vi "FTP Move_Status_Errors.vi"(8 "error in (no error)":errorcluster, 9 "Dir of file to FTP":path, 10 "FTP input cluster":T1={"Host"="", "UserName"="", "PassWord"="", "FTP File Path"="", "Timeout (S)"=0, "ActivePasive"=FALSE, "Binary Ascii"=FALSE, "Remote Port"=21} {"Timeout (S)" min=0 max=300 step=1}, 11 "File to Move":string) -> (1 "concatenated string of Error":string, 3 "FTP completed (true = good)":bool)   [LabVIEW 2011]
uses:
  Controls/FTP Credintials.ctl
  <vilib>/addons/internet/NI_InternetTK_FTP_VIs.lvlib
panel:
  # "Passive"
  # "Active"
  # "Binary"
  # "Ascii"
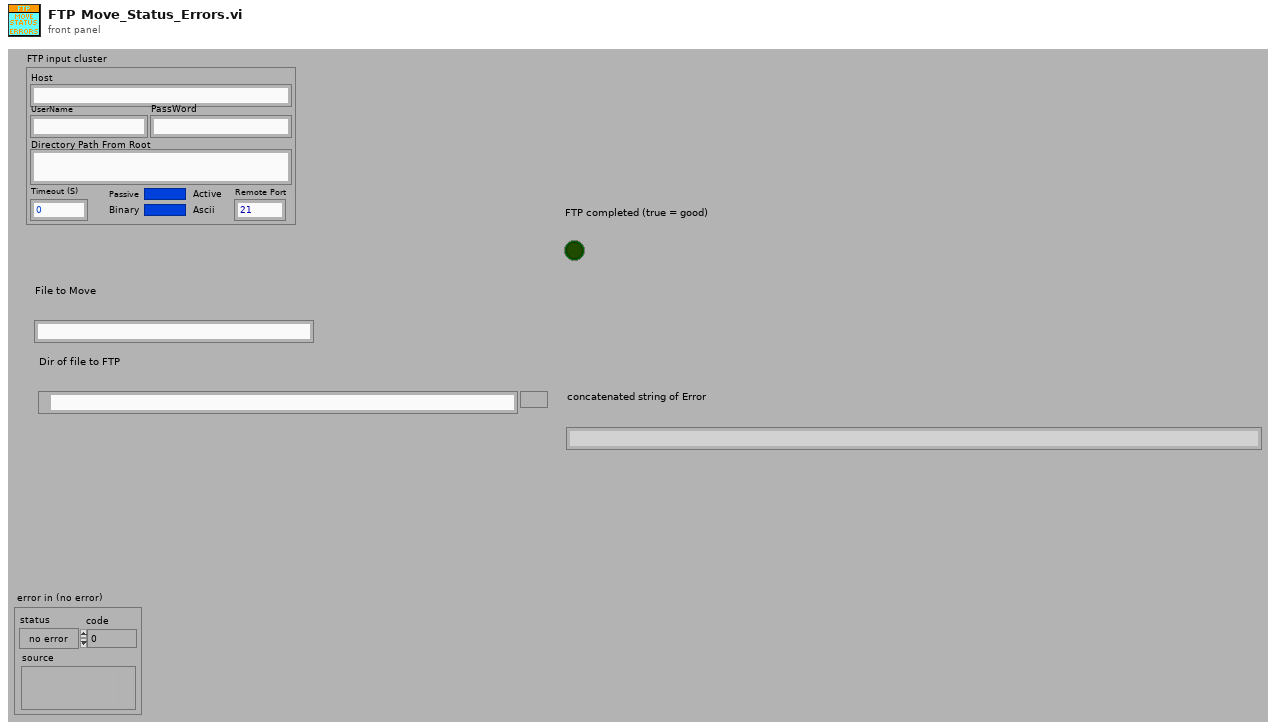
[diagram p1: front panel]
types:
  T1 = typedef "FTP Credintials.ctl" = cluster{"Host":string, "UserName":string, "PassWord":string, "FTP File Path":string, "Timeout (S)":i32, "ActivePasive":bool, "Binary Ascii":bool, "Remote Port":u16}
  T2 = typedef "FTP Session.ctl" = refnum<k1>
  T3 = cluster{string, "appended path":path, "Binary Ascii":bool, string}
  T4 = cluster{string, "appended path":path, "Binary Ascii":bool, string}[]
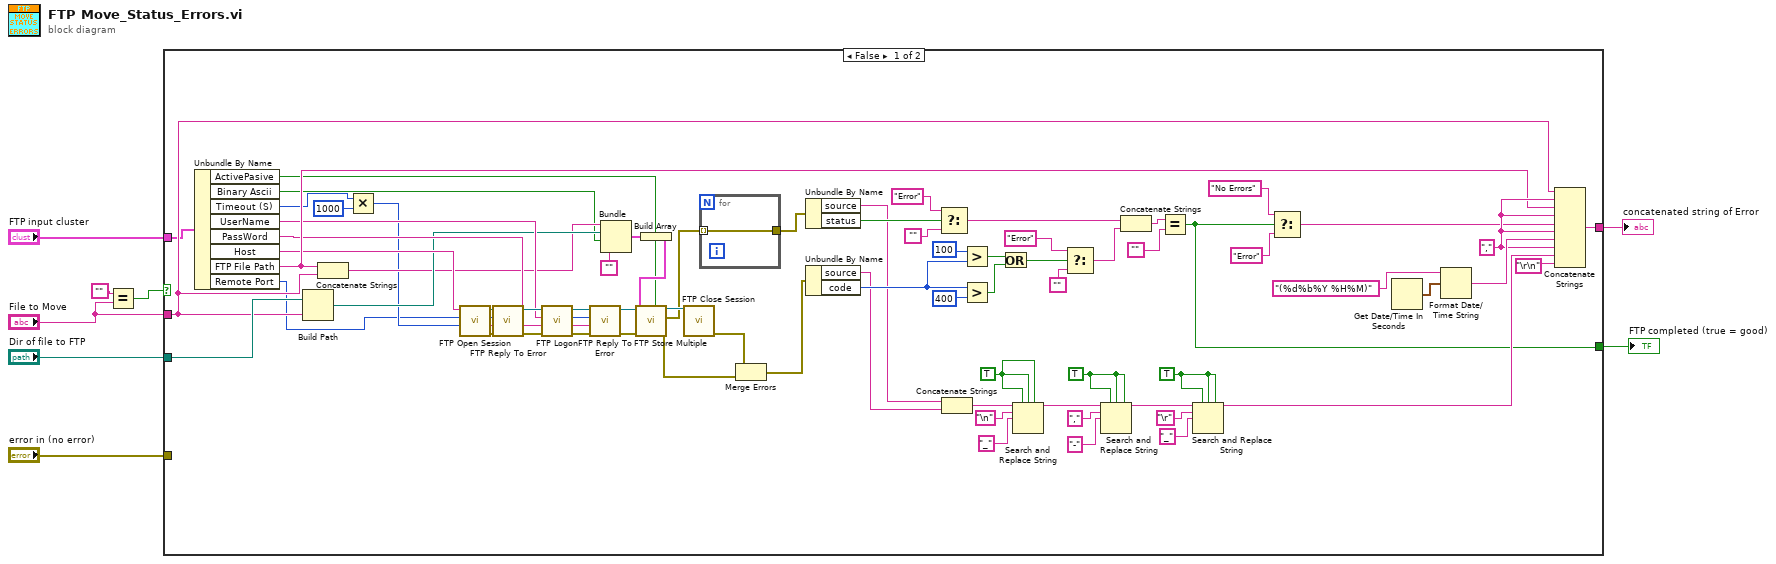
[diagram p0: block diagram]
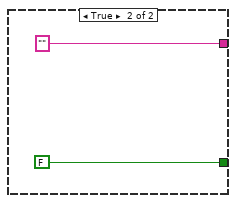
[diagram p2: hidden frame]
diagram:
  n1 = Equal?(x="", y="File to Move") -> (x = y?=w2:bool)
  n2 = case shown="False" w2 {
    tunnel: "Dir of file to FTP" -> [w68 _]
    tunnel: [w67 ""] -> w7
    tunnel: "File to Move" -> [w66 _]
    tunnel: "FTP input cluster" -> [w65 _]
    tunnel: [w12 FALSE] -> w6
    tunnel: "error in (no error)" -> [_ _]
    frame False {
      w60 = TRUE ("replace all? (F)")
      w59 = TRUE ("replace all? (F)")
      w50 = TRUE ("replace all? (F)")
      w70 = "," ("string")
      n3 = Unbundle By Name(w65) -> ("ActivePasive"=w10:bool, "Binary Ascii"=w11:bool, "Timeout (S)"=w21:i32, "UserName"=w31:string, "PassWord"=w32:string, "Host"=w33:string, "FTP File Path"=w69:string, "Remote Port"=w9:u16)
      n4 = Build Path(base path=w68, name or relative path=w66) -> (appended path=w30:path)
      n5 = Concatenate Strings(w69, w66) -> (w29:string)
      n6 = Multiply(x=w21, y=1000) -> (x*y=w22:i32)
      n7 = call <vilib>:"FTP Open Session.vi"("timeout ms (60000)"=w22, "remote port (21)"=w9, "address"=w33) -> ("error out"=w26:errorcluster, "reply string"=w39:string, "reply code"=w38:i32, "ftp session"=w37:T2)  [unwired: 1 in, 4 out]
      n8 = call <vilib>:"FTP Reply To Error.vi"("error in (no error)"=w26, "reply string in"=w39, "reply code in"=w38, "ftp session"=w37) -> ("error out"=w41:errorcluster, "ftp session out"=w40:T2)  [unwired: 2 out]
      n9 = call <vilib>:"FTP Logon.vi"("error in (no error)"=w41, "password"=w32, "user"=w31, "ftp session"=w40) -> ("error out"=w42:errorcluster, "reply string"=w45:string, "reply code"=w44:i32, "ftp session out"=w43:T2)  [unwired: 4 out]
      n10 = call <vilib>:"FTP Reply To Error.vi"("error in (no error)"=w42, "reply string in"=w45, "reply code in"=w44, "ftp session"=w43) -> ("error out"=w46:errorcluster, "ftp session out"=w47:T2)  [unwired: 2 out]
      n11 = Bundle(w29, "appended path"=w30, "Binary Ascii"=w11, "") -> (w35:T3)  [unwired: 1 out]
      n12 = Build Array(w35) -> (w34:T4)
      n13 = call <vilib>:"FTP Store Multiple.vi"("active (T)"=w10, "error in (no error)"=w46, "file specifications"=w34, "ftp session"=w47) -> ("error out"=w24:errorcluster, "file errors"=w28:errorcluster[], "ftp session out"=w48:T2)  [unwired: 5 out]
      n14 = call <vilib>:"FTP Close Session.vi"("ftp session"=w48) -> ("error out"=w25:errorcluster)  [unwired: 1 in, 9 out]
      n15 = for {
        tunnel: w28 -> [w85] mode=indexing
        tunnel: [w85] -> w27
      }
      n16 = Merge Errors(w25, w24) -> (w23:errorcluster)
      n17 = Unbundle By Name(w27) -> ("source"=w16:string, "status"=w64:bool)
      n18 = Unbundle By Name(w23) -> ("source"=w15:string, "code"=w74:i32)
      n19 = Select(t="Error", s=w64, f="") -> (s? t:f=w79:string)
      n20 = Concatenate Strings(w16, w15) -> (w17:string)
      n21 = Greater?(x=100, y=w74) -> (0:w72:bool)
      n22 = Greater?(x=w74, y=400 ("x")) -> (0:w75:bool)
      n23 = Or(x=w72, y=w75) -> (x .or. y?=w63:bool)
      n24 = Search and Replace String(replace all?=w50, case sensitive?=w50, multiline?=w50, input string=w17, search string="\n", replace string="_" ("replace string (\"\")")) -> (result string=w55:string)  [unwired: 2 in, 3 out]
      n25 = Select(t="Error", s=w63, f="") -> (s? t:f=w80:string)
      n26 = Search and Replace String(replace all?=w59, case sensitive?=w59, multiline?=w59, input string=w55, search string=",", replace string="-" ("replace string (\"\")")) -> (result string=w58:string)  [unwired: 2 in, 3 out]
      n27 = Concatenate Strings(w79, w80) -> (w77:string)
      n28 = Equal?(x=w77, y="") -> (x = y?=w12:bool)
      n29 = Search and Replace String(replace all?=w60, case sensitive?=w60, multiline?=w60, input string=w58, search string="\r", replace string="_" ("replace string (\"\")")) -> (result string=w49:string)  [unwired: 2 in, 3 out]
      n30 = Select(t="No Errors", s=w12, f="Error" ("t")) -> (s? t:f=w14:string)
      n31 = Get Date/Time In Seconds() -> (seconds since 1Jan1904=w84:timestamp)
      n32 = Format Date/Time String(time format string (%c)="(%d%b%Y %H%M)", seconds (now)=w84) -> (date/time string=w82:string)  [unwired: 1 in]
      n33 = Concatenate Strings(w66, w70, w69, w70, w14, w70, w82, w70, w49, "\r\n") -> (w67:string)
    }
    frame True {
    }
  }
  "concatenated string of Error" <- w7
  "FTP completed (true = good)" <- w6
